vi "Actor Template-Core_Process.vi"(0 "FTW Actor Instance Configuration":string="{\n  \"Identity\": \"ActorName\",\n  \"InboxAddress\": \"tcp://127.0.0.1:*\",\n  \"PublisherAddress\": \"tcp://127.0.0.1:*\",\n  \"DebugEnableInboxLogging\": false,\n  \"DebugEnableJobLogging\": false,\n  \"DebugShowPanel\": false\n}", 11 "ErrorIn":errorcluster) -> (15 "Error":errorcluster)   [LabVIEW 2012, in "Actor Template-Core.lvclass"]
uses:
  Actor Template-Core.lvclass
  src/Instance/FTW-ActorInstance.lvclass
  src/Message/Request/FTW-Message-IncomingRequest.lvclass
panel:
  # "#TODO\nhide controls for a GUI"
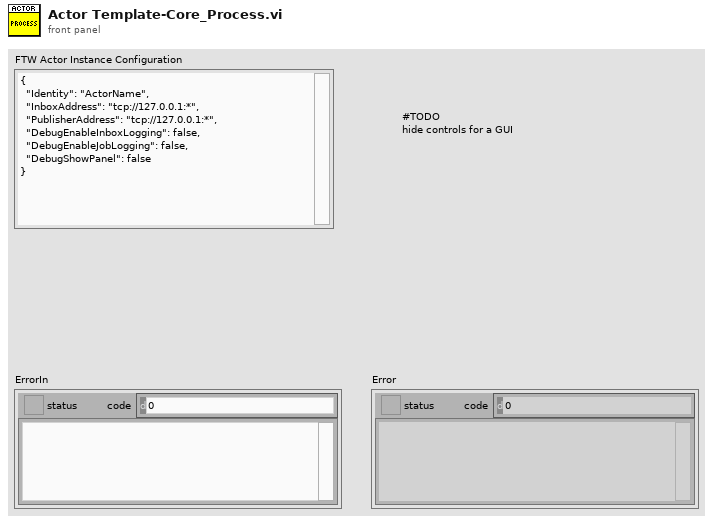
[diagram p1: front panel]
types:
  T1 = cluster{"Incoming Requests":refnum<event-registration>, "Additional Registration Types":refnum<event-registration>}
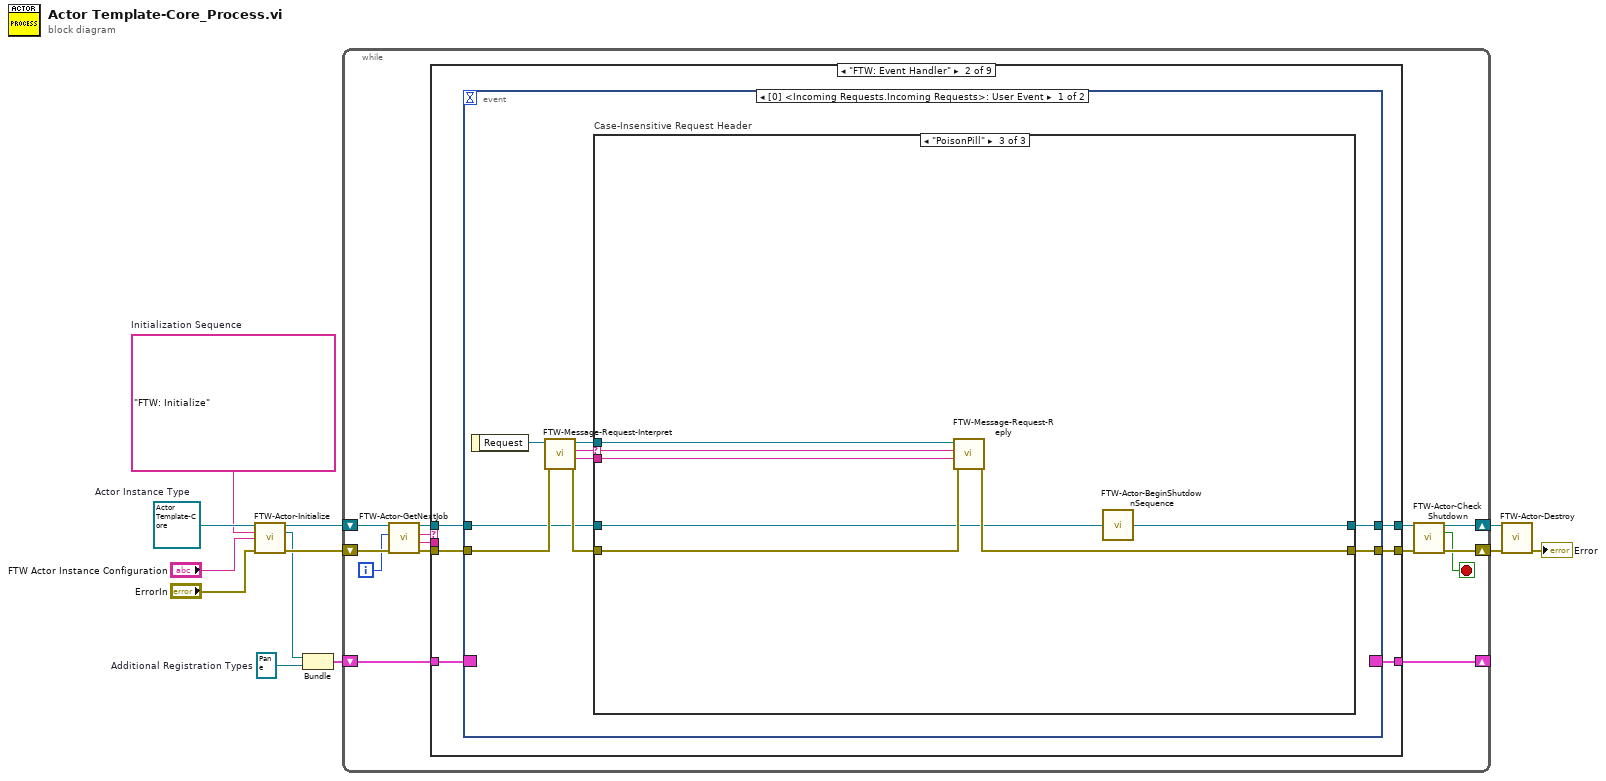
[diagram p0: block diagram]
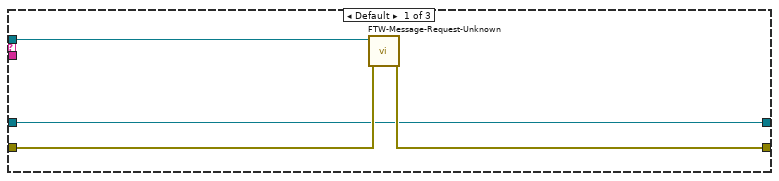
[diagram p3: hidden frame]
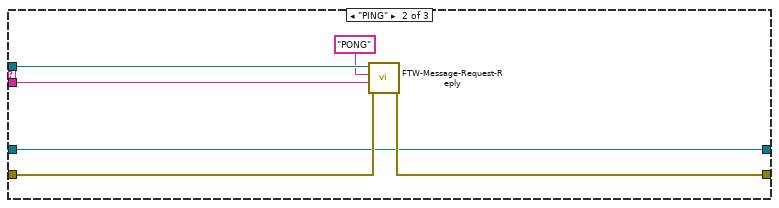
[diagram p4: hidden frame]
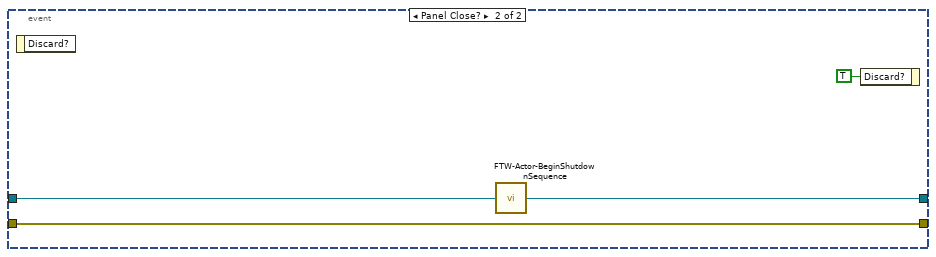
[diagram p5: hidden frame]
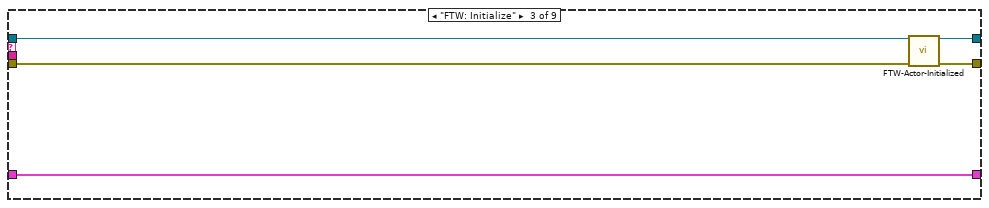
[diagram p6: hidden frame]
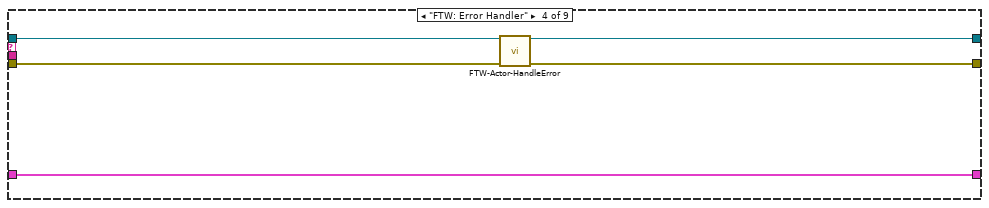
[diagram p7: hidden frame]
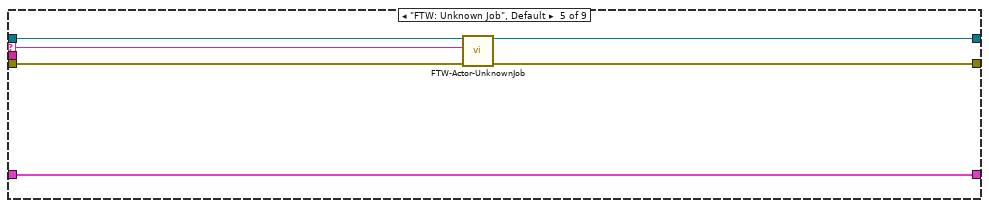
[diagram p8: hidden frame]
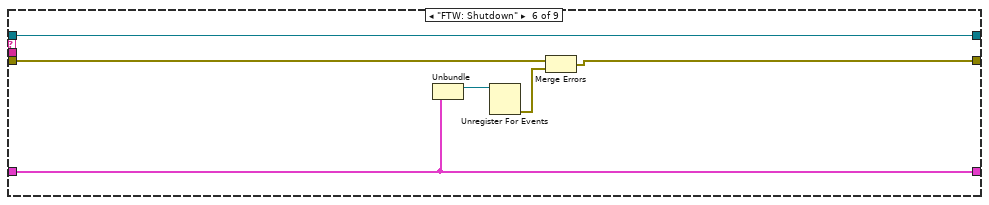
[diagram p9: hidden frame]
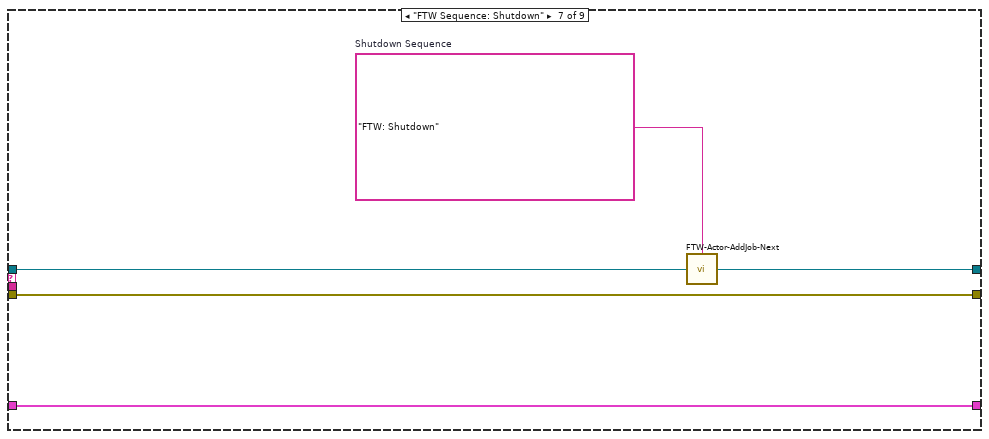
[diagram p10: hidden frame]
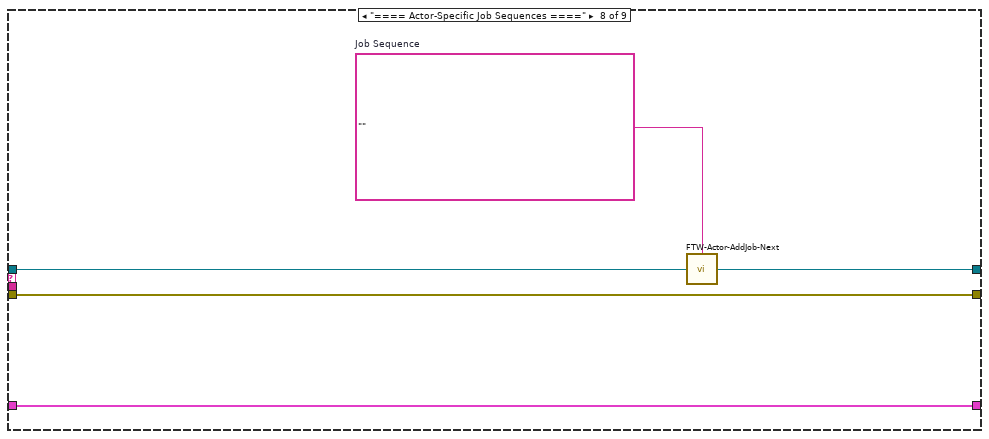
[diagram p11: hidden frame]
diagram:
  w4 = refnum<event-registration> refnum  # Additional Registration Types
  w7 = refnum<class "Actor Template-Core.lvclass"> refnum  # Actor Instance Type
  w6 = "FTW: Initialize"  # Initialization Sequence
  n1 = call-dynamic "FTW-Actor-Initialize.vi"("FTW Actor Instance Type"=w7, "Initialization Job Sequence"=w6, "Actor Instance Configuration"="FTW Actor Instance Configuration", "error in"="ErrorIn") -> ("FTW Actor Instance"=w12:refnum<class "Actor Template-Core.lvclass">, "Incoming Requests"=w1:refnum<event-registration>, "error out"=w8:errorcluster)  [unwired: 9 in]
  n2 = Bundle("Incoming Requests"=w1, "Additional Registration Types"=w4) -> (w3:T1)  [unwired: 1 in]
  n3 = while {
    shift-right: [w16] -> w10
    shift-left: w8 -> [w23]
    shift-right: [w13] -> _
    shift-left: w3 -> [w26]
    shift-right: [w18] -> w11
    shift-left: w12 -> [w25]
    i -> [w14]
    stop <- w15 stop-if-true
    n4 = call "FTW-Actor-GetNextJob.vi"("error in"=w23, "Jobs Performed"=w14, "FTW Actor Instance"=w25) -> ("error out"=w22:errorcluster, "Job Data"=w20:string, "Job Name"=w21:string, "FTW Actor Instance out"=w24:refnum<class "Actor Template-Core.lvclass">)  [unwired: 5 in]
    n5 = case shown="\"FTW: Event Handler\"" w21 {
      selector: w21 -> [_ _ _ _ w76 _ _ _ _]
      tunnel: [w28 w35 w66 w71 w79 w84 w91 w96 w100] -> w17
      tunnel: w22 -> [w28 w34 w69 w73 w80 w85 w91 w96 w100]
      tunnel: w26 -> [w29 w30 w70 w75 w81 w87 w92 w97 w99]
      tunnel: [w29 w33 w70 w75 w81 w87 w92 w97 w99] -> w13
      tunnel: w20 -> [_ _ _ _ _ _ _ _ _]
      tunnel: [w27 w32 w67 w72 w77 w82 w89 w94 w98] -> w19
      tunnel: w24 -> [w27 w31 w68 w74 w78 w82 w90 w95 w98]
      frame "==== Featherweight Framework Jobs ====" {
      }
      frame "FTW: Event Handler" {
        n6 = event shown="[0] <Incoming Requests.Incoming Requests>: User Event" {
          selector: w30 -> [_ _]
          dyn-events: [_ _] -> w33
          timeout: _ -> [_ _]
          tunnel: [w41 w64] -> w35
          tunnel: w34 -> [w42 w64]
          tunnel: [w40 w62] -> w32
          tunnel: w31 -> [w39 w63]
          event User Event {
            n7 = event-data() -> ("Request"=w43:refnum<class "FTW-Message-IncomingRequest.lvclass">)  [unwired: 1 in]
            n8 = call "FTW-Message-Request-Interpret.vi"("error in"=w42, "FTW Incoming Request"=w43) -> ("error out"=w44:errorcluster, "Request Body"=w37:string, "Request Header"=w38:string, "FTW Incoming Request out"=w36:refnum<class "FTW-Message-IncomingRequest.lvclass">)  [unwired: 6 in]
            n9 = case "Case-Insensitive Request Header" shown="\"PoisonPill\"" w38 {
              selector: w38 -> [_ _ w56]
              tunnel: [w47 w51 w58] -> w41
              tunnel: w44 -> [w48 w52 w59]
              tunnel: [w45 w49 w61] -> w40
              tunnel: w39 -> [w45 w49 w57]
              tunnel: w37 -> [_ w53 w55]
              tunnel: w36 -> [w46 w54 w60]
              frame Default {
                n10 = call "FTW-Message-Request-Unknown.vi"("error in"=w48, "FTW Incoming Request"=w46) -> ("error out"=w47:errorcluster)  [unwired: 9 in]
              }
              frame "PING" {
                n11 = call "FTW-Message-Request-Reply.vi"("error in"=w52, "Response Body"=w53, "Response Header"="PONG", "FTW Incoming Request"=w54) -> ("error out"=w51:errorcluster)  [unwired: 6 in, 1 out]
              }
              frame "PoisonPill" {
                n12 = call "FTW-Message-Request-Reply.vi"("error in"=w59, "Response Body"=w55, "Response Header"=w56, "FTW Incoming Request"=w60) -> ("error out"=w58:errorcluster)  [unwired: 6 in, 1 out]
                n13 = call "FTW-Actor-BeginShutdownSequence.vi"("FTW Actor Instance"=w57) -> ("FTW Actor Instance out"=w61:refnum<class "Actor Template-Core.lvclass">)  [unwired: 3 in]
              }
            }
          }
          event Panel Close? {
            n14 = event-data() -> ()  [unwired: 1 in, 1 out]
            n15 = call "FTW-Actor-BeginShutdownSequence.vi"("FTW Actor Instance"=w63) -> ("FTW Actor Instance out"=w62:refnum<class "Actor Template-Core.lvclass">)  [unwired: 3 in]
            n16 = event-data("Discard?"=TRUE) -> ()  [unwired: 1 in, 1 out]
          }
        }
      }
      frame "FTW: Initialize" {
        n17 = call-dynamic "FTW-Actor-Initialized.vi"("FTW Actor Instance"=w68, "error in"=w69) -> ("FTW Actor Instance out"=w67:refnum<class "Actor Template-Core.lvclass">, "error out"=w66:errorcluster)  [unwired: 12 in]
      }
      frame "FTW: Error Handler" {
        n18 = call-dynamic "FTW-Actor-HandleError.vi"("FTW Actor Instance"=w74, "error in"=w73) -> ("FTW Actor Instance out"=w72:refnum<class "Actor Template-Core.lvclass">, "error out"=w71:errorcluster)  [unwired: 11 in, 1 out]
      }
      frame "FTW: Unknown Job", Default {
        n19 = call-dynamic "FTW-Actor-UnknownJob.vi"("FTW Actor Instance"=w78, "Unknown Job"=w76, "error in"=w80) -> ("FTW Actor Instance out"=w77:refnum<class "Actor Template-Core.lvclass">, "error out"=w79:errorcluster)  [unwired: 11 in]
      }
      frame "FTW: Shutdown" {
        n20 = Unbundle(w87) -> ("Incoming Requests"=w86:refnum<event-registration>)  [unwired: 1 out]
        n21 = Unregister For Events(event registration refnum=w86) -> (error out=w83:errorcluster)  [unwired: 1 in]
        n22 = Merge Errors(w85, w83) -> (w84:errorcluster)
      }
      frame "FTW Sequence: Shutdown" {
        w88 = "FTW: Shutdown"  # Shutdown Sequence
        n23 = call "FTW-Actor-AddJob-Next.vi"("Add Next in Job Queue"=w88, "FTW Actor Instance"=w90) -> ("FTW Actor Instance out"=w89:refnum<class "Actor Template-Core.lvclass">)  [unwired: 2 in]
      }
      frame "==== Actor-Specific Job Sequences ====" {
        w93 = ""  # Job Sequence
        n24 = call "FTW-Actor-AddJob-Next.vi"("Add Next in Job Queue"=w93, "FTW Actor Instance"=w95) -> ("FTW Actor Instance out"=w94:refnum<class "Actor Template-Core.lvclass">)  [unwired: 2 in]
      }
      frame "==== Actor-Specific Jobs ====" {
      }
    }
    n25 = call "FTW-Actor-CheckShutdown.vi"("FTW Actor Instance"=w19, "error in"=w17) -> ("FTW Actor Instance out"=w18:refnum<class "Actor Template-Core.lvclass">, "Shutdown?"=w15:bool, "error out"=w16:errorcluster)  [unwired: 11 in]
  }
  n26 = call-dynamic "FTW-Actor-Destroy.vi"("FTW Actor Instance"=w11, "error in"=w10) -> ("error out"=→"Error":errorcluster)  [unwired: 13 in]
